vi "To String.vi"(8 "error in (no error)":errorcluster, 11 "bytes in":refnum<class "bytes.lvclass">) -> (0 "error out":errorcluster, 2 "String":string, 3 "bytes out":refnum<class "bytes.lvclass">)   [LabVIEW 2020, in "Protobuf RAW.lvlib" / "bytes.lvclass"]
uses:
  bytes.lvclass
  bytes.lvclass/bytes.ctl
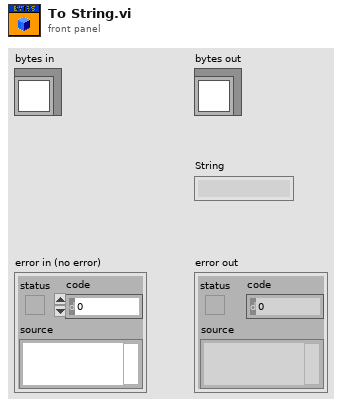
[diagram p1: front panel]
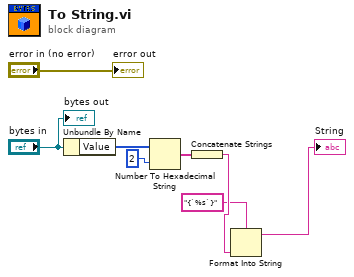
[diagram p0: block diagram]
diagram:
  n1 = Unbundle By Name("bytes in") -> ("Value"=w7:u8[])
  n2 = Number To Hexadecimal String(1:i16 2 ("width (-)"), 2:w7) -> (0:w5:string[])
  n3 = Concatenate Strings(w5) -> (w3:string)
  n4 = Format Into String(format string="{`%s`}", w3) -> (resulting string=→"String":string)  [unwired: 2 in, 1 out]
  "error out" <- "error in (no error)"
  "bytes out" <- "bytes in"
